vi "Start (Unconfigured).vi"(8 "error in (no error)":errorcluster, 11 "Volatus Core in":refnum<class "Volatus Core.lvclass">) -> (0 "error out":errorcluster, 2 "MessageQ":refnum<class "MessageQ.lvclass">)   [LabVIEW 2020, in "Volatus.lvlib" / "Volatus Core.lvclass"]
uses:
  Volatus Core.lvclass
  Volatus Core.lvclass/Volatus Core.ctl
  Config Type.ctl
  MessageQ/MessageQ.lvclass
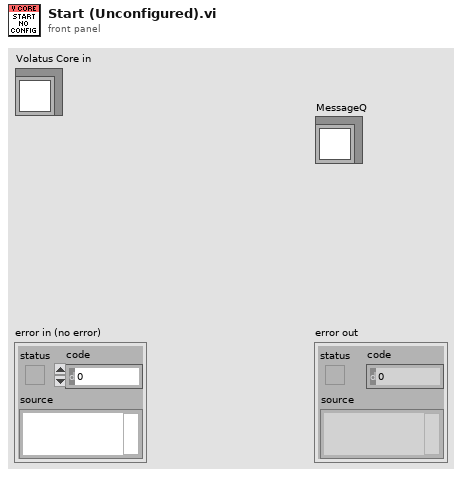
[diagram p1: front panel]
types:
  T1 = typedef "Volatus.lvlib/Volatus Core.lvclass/Config Type.ctl" = enum16{"App INI", "Memory", "Unconfigured"}
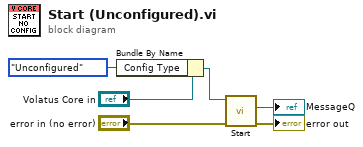
[diagram p0: block diagram]
diagram:
  n1 = Bundle By Name(cluster="Volatus Core in", "Config Type"=Config_Type."Unconfigured") -> (w3:refnum<class "Volatus Core.lvclass">)
  n2 = call "Start.vi"("error in (no error)"="error in (no error)", "Volatus Core in"=w3) -> ("error out"=→"error out":errorcluster, "MessageQ"=→"MessageQ":refnum<class "MessageQ.lvclass">)  [unwired: 8 in]
